vi "multimetro.vi"(8 "error in (no error)":errorcluster, 11 "mediciones":i32) -> (0 "error out":errorcluster, 1 "voltajeProm":dbl, 2 "voltaje":dbl)   [LabVIEW 2018]
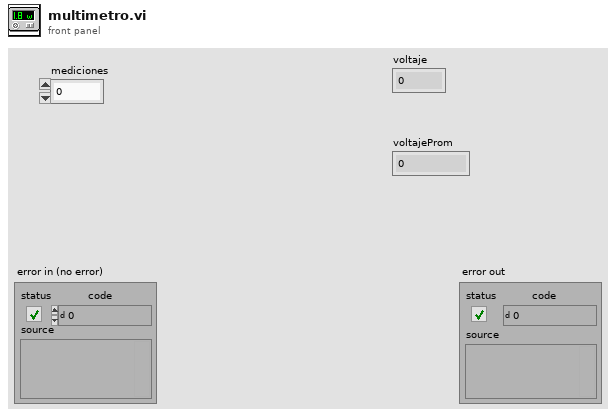
[diagram p1: front panel]
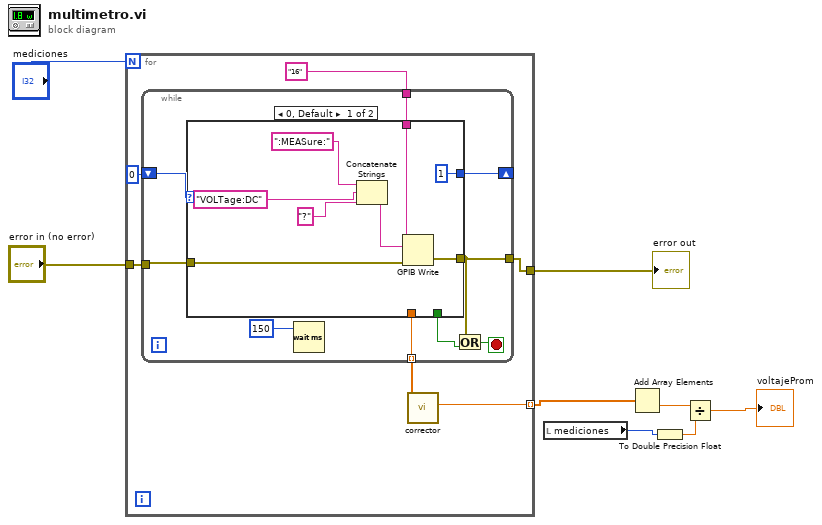
[diagram p0: block diagram]
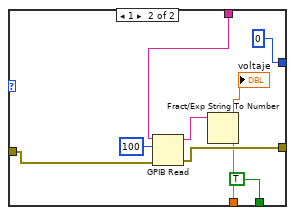
[diagram p2: hidden frame]
diagram:
  n1 = for {
    N: "mediciones" -> [_]
    tunnel: "error in (no error)" -> [w14]
    tunnel: [w11] -> w7
    tunnel: [w9] -> w4 mode=indexing
    n2 = while {
      tunnel: w14 -> [w22]
      shift-right: [w15] -> _
      shift-left: 0 -> [w23]
      tunnel: [w18] -> w11
      tunnel: "16" -> [w21]
      tunnel: [w16] -> w10 mode=indexing
      stop <- w19 stop-if-true
      n3 = case shown="0, Default" w23 {
        tunnel: w22 -> [w27 w36]
        tunnel: [w26 w35] -> w18
        tunnel: w21 -> [w25 w37]
        tunnel: [_ TRUE] -> w17
        tunnel: [_ w33] -> w16
        tunnel: [1 0] -> w15
        frame 0, Default {
          n4 = Concatenate Strings(":MEASure:" ("string"), "VOLTage:DC", "?" ("string")) -> (w28:string)
          n5 = GPIB Write(0:w25, 1:w28, 3:w27) -> (6:w26:errorcluster)  [unwired: 2 in, 1 out]
        }
        frame 1 {
          n6 = GPIB Read(0:w37, 1:100 ("byte count"), 3:w36) -> (5:w38:string, 7:w35:errorcluster)  [unwired: 2 in, 1 out]
          n7 = Fract/Exp String To Number(string=w38) -> (number=w33:dbl)  [unwired: 3 in, 1 out]
          "voltaje" <- w33
        }
      }
      n8 = Wait (ms)(milliseconds to wait=u32 150) -> ()  [unwired: 1 out]
      n9 = Or(x=w18, y=w17) -> (x .or. y?=w19:bool)
    }
    n10 = call "corrector.vi"("Array"=w10) -> ("valor salida"=w9:dbl)  [unwired: 10 in]
  }
  "error out" <- w7
  n11 = local read "mediciones"() -> (w2:i32)
  n12 = Add Array Elements(numeric array=w4) -> (sum=w6:dbl)
  n13 = To Double Precision Float(number=w2) -> (double precision float=w5:dbl)
  n14 = Divide(x=w6, y=w5) -> (x/y=→"voltajeProm":dbl)
